vi "Custom Symbols.vi"() -> (2 "Custom symbols":T1[](array[typedef])=[{"image type"=0, "image depth"=32, "image"=[0, 0, 0, 0, 0, 0, 0, 0, 0, 0, 0, 0, 0, 0, 0, 0, 0, 0, 0, 0, 0, 0, 0, 0, 0, 0, 0, 0, 0, 0, 0, 0, 0, 0, 0, 0, 0, 0, 0, 0, 0, 0, 0, 0, 0, 0, 0, 0, 0, 0, 0, 0, 0, 0, 0, 0, 0, 0, 0, 0, 0, 0, 0, 0, 0, 0, 0, 0, 0, 0, 0, 0, 0, 0, 0, 0, 0, 0, 0, 0, 0, 0, 0, 0, 0, 0, 0, 0, 0, 0, 0, 0, 0, 0, 0, 0, 0, 0, 0, 0, 0, 0, 0, 0, 0, 0, 0, 0, 0, 0, 0, 0, 0, 0, 0, 0, 0, 0, 0, 0, 0, 0, 0, 0, 0, 0, 0, 0, 0, 0, 0, 0, 0, 0, 0, 0, 0, 0, 0, 0, 0, 0, 0, 0, 0, 0, 0, 0, 0, 0, 0, 0, 0, 0, 0, 0, 0, 0, 0, 0, 0, 0, 0, 0, 0, 0, 0, 0, 0, 0, 0, 0, 0, 0, 0, 0, 0, 0, 0, 0, 0, 0, 0, 0, 0, 0, 0, 0, 0, 0, 0, 0, 0, 0, 0, 0, 0, 0, 0, 0, 0, 0, 0, 0, 0, 0, 0, 0, 0, 0, 0, 0, 0, 0, 0, 0, 0, 0, 0, 0, 0, 0, 0, 0, 0, 0, 0, 0, 255, 66, 161, 255, 255, 64, 156, 255, 0, 0, 0, 0, 0, 0, 0, 0, 0, 0, 0, 0, 0, 0, 0, 0, 0, 0, 0, 0, 0, 0, 0, 0, 0, 0, 0, 0, 0, 0, 0, 0, 0, 0, 0, 0, 0, 0, 0, 0, 0, 0, 0, 0, 0, 0, 0, 0, 0, 0, 0, 0, 0, 0, 0, 0, 255, 57, 140, 255, 255, 65, 158, 255, 255, 54, 131, 255, 0, 0, 0, 0, 0, 0, 0, 0, 0, 0, 0, 0, 0, 0, 0, 0, 0, 0, 0, 0, 0, 0, 0, 0, 0, 0, 0, 0, 0, 0, 0, 0, 0, 0, 0, 0, 0, 0, 0, 0, 0, 0, 0, 0, 0, 0, 0, 0, 0, 0, 0, 0, 255, 56, 138, 255, 255, 58, 142, 255, 255, 52, 128, 255, 255, 44, 107, 238, 0, 0, 0, 0, 0, 0, 0, 0, 0, 0, 0, 0, 0, 0, 0, 0, 0, 0, 0, 0, 255, 64, 156, 255, 255, 60, 146, 255, 255, 59, 144, 255, 255, 59, 144, 255, 255, 58, 142, 255, 0, 0, 0, 0, 0, 0, 0, 0, 255, 62, 151, 255, 255, 56, 138, 255, 255, 52, 126, 255, 255, 47, 115, 255, 255, 44, 107, 237, 0, 0, 0, 0, 0, 0, 0, 0, 0, 0, 0, 0, 255, 57, 140, 255, 255, 65, 159, 255, 255, 62, 151, 255, 255, 60, 147, 255, 255, 60, 147, 255, 255, 57, 141, 255, 0, 0, 0, 0, 0, 0, 0, 0, 255, 63, 154, 255, 255, 58, 141, 255, 255, 51, 124, 255, 255, 48, 117, 255, 255, 47, 115, 255, 255, 44, 107, 236, 0, 0, 0, 0, 0, 0, 0, 0, 255, 51, 124, 255, 255, 57, 140, 255, 255, 54, 133, 255, 255, 52, 127, 255, 255, 51, 126, 255, 255, 47, 116, 255, 0, 0, 0, 0, 0, 0, 0, 0, 255, 57, 139, 255, 255, 56, 137, 255, 255, 50, 123, 255, 255, 47, 116, 255, 255, 46, 112, 248, 255, 43, 105, 233, 0, 0, 0, 0, 0, 0, 0, 0, 0, 0, 0, 0, 255, 51, 125, 255, 255, 45, 110, 245, 255, 42, 102, 226, 255, 41, 101, 224, 255, 38, 93, 207, 0, 0, 0, 0, 0, 0, 0, 0, 255, 45, 110, 245, 255, 50, 123, 255, 255, 50, 122, 255, 255, 45, 110, 244, 255, 40, 97, 216, 0, 0, 0, 0, 0, 0, 0, 0, 0, 0, 0, 0, 0, 0, 0, 0, 0, 0, 0, 0, 0, 0, 0, 0, 0, 0, 0, 0, 0, 0, 0, 0, 0, 0, 0, 0, 0, 0, 0, 0, 0, 0, 0, 0, 255, 40, 97, 215, 255, 50, 121, 255, 255, 48, 118, 255, 255, 40, 97, 215, 0, 0, 0, 0, 0, 0, 0, 0, 0, 0, 0, 0, 0, 0, 0, 0, 0, 0, 0, 0, 0, 0, 0, 0, 0, 0, 0, 0, 0, 0, 0, 0, 0, 0, 0, 0, 0, 0, 0, 0, 0, 0, 0, 0, 0, 0, 0, 0, 255, 41, 100, 221, 255, 52, 126, 255, 255, 43, 106, 235, 0, 0, 0, 0, 0, 0, 0, 0, 0, 0, 0, 0, 0, 0, 0, 0, 0, 0, 0, 0, 0, 0, 0, 0, 0, 0, 0, 0, 0, 0, 0, 0, 0, 0, 0, 0, 0, 0, 0, 0, 0, 0, 0, 0, 0, 0, 0, 0, 0, 0, 0, 0, 255, 45, 110, 245, 255, 49, 121, 255, 0, 0, 0, 0, 0, 0, 0, 0, 0, 0, 0, 0, 0, 0, 0, 0, 0, 0, 0, 0, 0, 0, 0, 0, 0, 0, 0, 0, 0, 0, 0, 0, 0, 0, 0, 0, 0, 0, 0, 0, 0, 0, 0, 0, 0, 0, 0, 0, 0, 0, 0, 0, 0, 0, 0, 0, 0, 0, 0, 0, 0, 0, 0, 0, 0, 0, 0, 0, 0, 0, 0, 0, 0, 0, 0, 0, 0, 0, 0, 0, 0, 0, 0, 0, 0, 0, 0, 0, 0, 0, 0, 0, 0, 0, 0, 0, 0, 0, 0, 0, 0, 0, 0, 0, 0, 0, 0, 0, 0, 0, 0, 0, 0, 0, 0, 0, 0, 0, 0, 0, 0, 0, 0, 0, 0, 0, 0, 0, 0, 0, 0, 0, 0, 0, 0, 0, 0, 0, 0, 0, 0, 0, 0, 0, 0, 0, 0, 0, 0, 0, 0, 0, 0, 0, 0, 0, 0, 0, 0, 0, 0, 0, 0, 0, 0, 0, 0, 0, 0, 0, 0, 0, 0, 0, 0, 0, 0, 0, 0, 0, 0, 0, 0, 0, 0, 0, 0, 0, 0, 0, 0, 0, 0, 0, 0, 0, 0, 0, 0, 0, 0, 0, 0, 0, 0, 0, 0, 0, 0, 0, 0, 0], "mask"=[0, 0, 0, 0, 0, 0, 0, 96, 0, 112, 0, 120, 62, 124, 126, 126, 126, 126, 62, 124, 0, 120, 0, 112, 0, 96, 0, 0, 0, 0, 0, 0], "colors"=[], "Rectangle"={"left"=0, "top"=0, "right"=16, "bottom"=16}}])   [LabVIEW 2020, in "VolatusGUI.lvlib" / "Telemetry Command Module.lvclass"]
uses:
  Telemetry Command Module.lvclass
  Telemetry Command Module.lvclass/Telemetry Command Module.ctl
  <vilib>/picture/picture.llb/imagedata.ctl
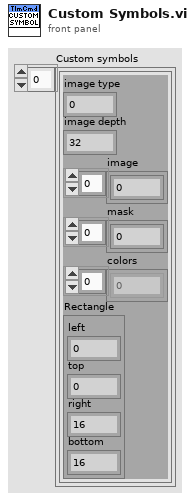
[diagram p1: front panel]
types:
  T1 = typedef "imagedata.ctl" = cluster{"image type":i32, "image depth":i32, "image":u8[], "mask":u8[], "colors":u32[], "Rectangle":cluster{"left":i16, "top":i16, "right":i16, "bottom":i16}}
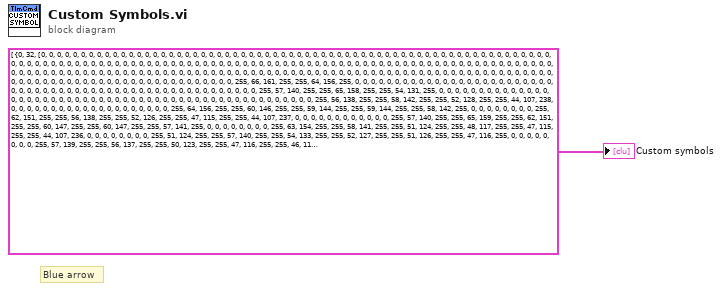
[diagram p0: block diagram]
diagram:
  # "Blue arrow"
  "Custom symbols" <- T1[] [{"image type"=0, "image depth"=32, "image"=[0, 0, 0, 0, 0, 0, 0, 0, 0, 0, 0, 0, 0, 0, 0, 0, 0, 0, 0, 0, 0, 0, 0, 0, 0, 0, 0, 0, 0, 0, 0, 0, 0, 0, 0, 0, 0, 0, 0, 0, 0, 0, 0, 0, 0, 0, 0, 0, 0, 0, 0, 0, 0, 0, 0, 0, 0, 0, 0, 0, 0, 0, 0, 0, 0, 0, 0, 0, 0, 0, 0, 0, 0, 0, 0, 0, 0, 0, 0, 0, 0, 0, 0, 0, 0, 0, 0, 0, 0, 0, 0, 0, 0, 0, 0, 0, 0, 0, 0, 0, 0, 0, 0, 0, 0, 0, 0, 0, 0, 0, 0, 0, 0, 0, 0, 0, 0, 0, 0, 0, 0, 0, 0, 0, 0, 0, 0, 0, 0, 0, 0, 0, 0, 0, 0, 0, 0, 0, 0, 0, 0, 0, 0, 0, 0, 0, 0, 0, 0, 0, 0, 0, 0, 0, 0, 0, 0, 0, 0, 0, 0, 0, 0, 0, 0, 0, 0, 0, 0, 0, 0, 0, 0, 0, 0, 0, 0, 0, 0, 0, 0, 0, 0, 0, 0, 0, 0, 0, 0, 0, 0, 0, 0, 0, 0, 0, 0, 0, 0, 0, 0, 0, 0, 0, 0, 0, 0, 0, 0, 0, 0, 0, 0, 0, 0, 0, 0, 0, 0, 0, 0, 0, 0, 0, 0, 0, 0, 0, 255, 66, 161, 255, 255, 64, 156, 255, 0, 0, 0, 0, 0, 0, 0, 0, 0, 0, 0, 0, 0, 0, 0, 0, 0, 0, 0, 0, 0, 0, 0, 0, 0, 0, 0, 0, 0, 0, 0, 0, 0, 0, 0, 0, 0, 0, 0, 0, 0, 0, 0, 0, 0, 0, 0, 0, 0, 0, 0, 0, 0, 0, 0, 0, 255, 57, 140, 255, 255, 65, 158, 255, 255, 54, 131, 255, 0, 0, 0, 0, 0, 0, 0, 0, 0, 0, 0, 0, 0, 0, 0, 0, 0, 0, 0, 0, 0, 0, 0, 0, 0, 0, 0, 0, 0, 0, 0, 0, 0, 0, 0, 0, 0, 0, 0, 0, 0, 0, 0, 0, 0, 0, 0, 0, 0, 0, 0, 0, 255, 56, 138, 255, 255, 58, 142, 255, 255, 52, 128, 255, 255, 44, 107, 238, 0, 0, 0, 0, 0, 0, 0, 0, 0, 0, 0, 0, 0, 0, 0, 0, 0, 0, 0, 0, 255, 64, 156, 255, 255, 60, 146, 255, 255, 59, 144, 255, 255, 59, 144, 255, 255, 58, 142, 255, 0, 0, 0, 0, 0, 0, 0, 0, 255, 62, 151, 255, 255, 56, 138, 255, 255, 52, 126, 255, 255, 47, 115, 255, 255, 44, 107, 237, 0, 0, 0, 0, 0, 0, 0, 0, 0, 0, 0, 0, 255, 57, 140, 255, 255, 65, 159, 255, 255, 62, 151, 255, 255, 60, 147, 255, 255, 60, 147, 255, 255, 57, 141, 255, 0, 0, 0, 0, 0, 0, 0, 0, 255, 63, 154, 255, 255, 58, 141, 255, 255, 51, 124, 255, 255, 48, 117, 255, 255, 47, 115, 255, 255, 44, 107, 236, 0, 0, 0, 0, 0, 0, 0, 0, 255, 51, 124, 255, 255, 57, 140, 255, 255, 54, 133, 255, 255, 52, 127, 255, 255, 51, 126, 255, 255, 47, 116, 255, 0, 0, 0, 0, 0, 0, 0, 0, 255, 57, 139, 255, 255, 56, 137, 255, 255, 50, 123, 255, 255, 47, 116, 255, 255, 46, 112, 248, 255, 43, 105, 233, 0, 0, 0, 0, 0, 0, 0, 0, 0, 0, 0, 0, 255, 51, 125, 255, 255, 45, 110, 245, 255, 42, 102, 226, 255, 41, 101, 224, 255, 38, 93, 207, 0, 0, 0, 0, 0, 0, 0, 0, 255, 45, 110, 245, 255, 50, 123, 255, 255, 50, 122, 255, 255, 45, 110, 244, 255, 40, 97, 216, 0, 0, 0, 0, 0, 0, 0, 0, 0, 0, 0, 0, 0, 0, 0, 0, 0, 0, 0, 0, 0, 0, 0, 0, 0, 0, 0, 0, 0, 0, 0, 0, 0, 0, 0, 0, 0, 0, 0, 0, 0, 0, 0, 0, 255, 40, 97, 215, 255, 50, 121, 255, 255, 48, 118, 255, 255, 40, 97, 215, 0, 0, 0, 0, 0, 0, 0, 0, 0, 0, 0, 0, 0, 0, 0, 0, 0, 0, 0, 0, 0, 0, 0, 0, 0, 0, 0, 0, 0, 0, 0, 0, 0, 0, 0, 0, 0, 0, 0, 0, 0, 0, 0, 0, 0, 0, 0, 0, 255, 41, 100, 221, 255, 52, 126, 255, 255, 43, 106, 235, 0, 0, 0, 0, 0, 0, 0, 0, 0, 0, 0, 0, 0, 0, 0, 0, 0, 0, 0, 0, 0, 0, 0, 0, 0, 0, 0, 0, 0, 0, 0, 0, 0, 0, 0, 0, 0, 0, 0, 0, 0, 0, 0, 0, 0, 0, 0, 0, 0, 0, 0, 0, 255, 45, 110, 245, 255, 49, 121, 255, 0, 0, 0, 0, 0, 0, 0, 0, 0, 0, 0, 0, 0, 0, 0, 0, 0, 0, 0, 0, 0, 0, 0, 0, 0, 0, 0, 0, 0, 0, 0, 0, 0, 0, 0, 0, 0, 0, 0, 0, 0, 0, 0, 0, 0, 0, 0, 0, 0, 0, 0, 0, 0, 0, 0, 0, 0, 0, 0, 0, 0, 0, 0, 0, 0, 0, 0, 0, 0, 0, 0, 0, 0, 0, 0, 0, 0, 0, 0, 0, 0, 0, 0, 0, 0, 0, 0, 0, 0, 0, 0, 0, 0, 0, 0, 0, 0, 0, 0, 0, 0, 0, 0, 0, 0, 0, 0, 0, 0, 0, 0, 0, 0, 0, 0, 0, 0, 0, 0, 0, 0, 0, 0, 0, 0, 0, 0, 0, 0, 0, 0, 0, 0, 0, 0, 0, 0, 0, 0, 0, 0, 0, 0, 0, 0, 0, 0, 0, 0, 0, 0, 0, 0, 0, 0, 0, 0, 0, 0, 0, 0, 0, 0, 0, 0, 0, 0, 0, 0, 0, 0, 0, 0, 0, 0, 0, 0, 0, 0, 0, 0, 0, 0, 0, 0, 0, 0, 0, 0, 0, 0, 0, 0, 0, 0, 0, 0, 0, 0, 0, 0, 0, 0, 0, 0, 0, 0, 0, 0, 0, 0, 0], "mask"=[0, 0, 0, 0, 0, 0, 0, 96, 0, 112, 0, 120, 62, 124, 126, 126, 126, 126, 62, 124, 0, 120, 0, 112, 0, 96, 0, 0, 0, 0, 0, 0], "colors"=[], "Rectangle"={"left"=0, "top"=0, "right"=16, "bottom"=16}}]
